vi "LVITX AddLetter.vi"(1 "String":string) -> (0 "output string":string)   [LabVIEW 2011]
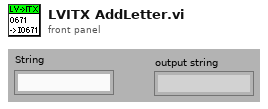
[diagram p1: front panel]
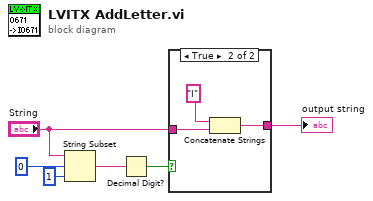
[diagram p0: block diagram]
diagram:
  n1 = String Subset(string="String", offset (0)=0, length (rest)=1 ("length (rest)")) -> (substring=w4:string)
  n2 = Decimal Digit?(1:w4) -> (0:w3:bool)
  n3 = case shown="True" w3 {
    tunnel: "String" -> [w7 w10]
    tunnel: [w7 w8] -> w1
    frame False {
    }
    frame True {
      n4 = Concatenate Strings("I", w10) -> (w8:string)
    }
  }
  "output string" <- w1
